vi "Initialize Listbox.vi"(5 "remove":refnum<vi>, 7 "add":refnum<vi>, 8 "error in (no error)":errorcluster, 9 "Names":string[](array[string]), 10 "Listbox":refnum<vi>, 11 "Item Ref":T2=18446744073709551615 format="%.0x") -> (0 "error out":errorcluster, 3 "Listbox Refs":T1 {"Section Ref" format="%.0x"})   [LabVIEW 2016, in "FPGA Addon System Explorer.lvlib"]
uses:
  FPGA Addon System Explorer.lvlib
  <vilib>/NI Veristand/Custom Device API/Custom Device Item Ref.ctl
  Listbox Cluster.ctl
  <vilib>/NI VeriStand/Custom Device API/Custom Device API.lvlib
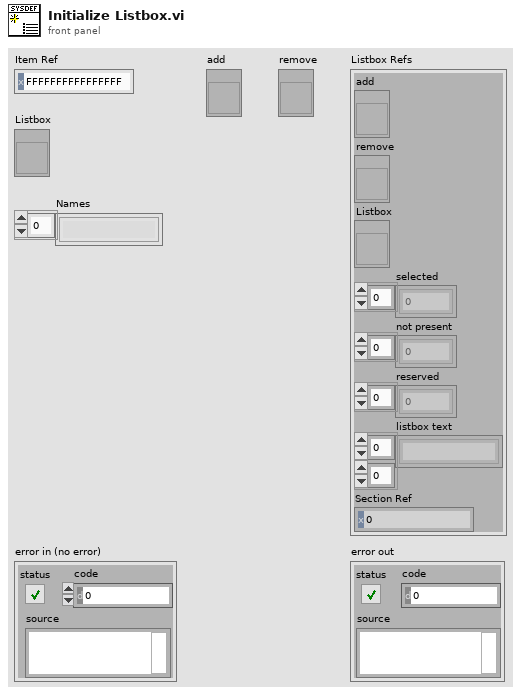
[diagram p1: front panel]
types:
  T1 = typedef "FPGA Addon System Explorer.lvlib/Listbox Cluster.ctl" = cluster{"add":refnum<vi>, "remove":refnum<vi>, "Listbox":refnum<vi>, "selected":i32[], "not present":i32[], "reserved":i32[], "listbox text":string[][], "Section Ref":T2}
  T2 = typedef "Custom Device API.lvlib/Custom Device Item Ref.ctl" = u64
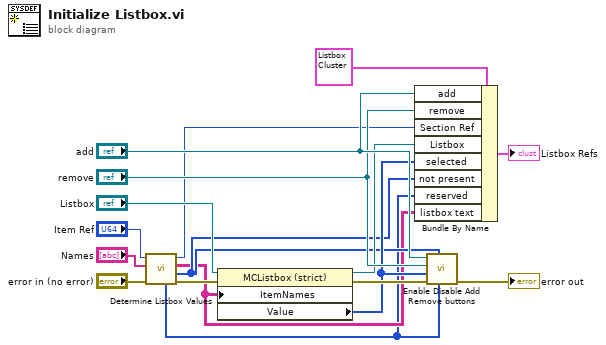
[diagram p0: block diagram]
diagram:
  n1 = call "Determine Listbox Values.vi"("error in (no error)"="error in (no error)", "List of Objects"="Names", "Section Ref in"="Item Ref") -> ("error out"=w13:errorcluster, "not present item indexes"=w4:i32[], "listbox text"=w3:string[][], "Section Ref out"=w7:T2, "reserved item indexes"=w1:i32[])  [unwired: 4 in]
  n2 = property class="MCListbox (strict)"(reference="Listbox", error in=w13, "ItemNames"=w3) -> (reference out=w6:refnum<vi>, error out=w17:errorcluster, "Value"=w5:i32[])
  n3 = Bundle By Name(cluster=T1 {"add"=refnum, "remove"=refnum, "Listbox"=refnum, "selected"=[], "not present"=[], "reserved"=[], "listbox text"=[], "Section Ref"=0}, "add"="add", "remove"="remove", "Section Ref"=w7, "Listbox"=w6, "selected"=w5, "not present"=w4, "reserved"=w1, "listbox text"=w3) -> (→"Listbox Refs":T1)
  n4 = call "Enable Disable Add Remove buttons.vi"("reserved item indexes"=w1, "not present item indexes"=w4, "error in (no error)"=w17, "selected items"=w5, "remove button"="remove", "add button"="add") -> ("error out"=→"error out":errorcluster)  [unwired: 5 in]
